vi "Calc Safe Reports.vi"(8 "tolerate 1 bad level?":bool, 9 "lower limit":i32, 10 "upper limit":i32, 11 "Reports":cluster{i32[]}[](array[cluster])) -> (3 "safe reports":u32)   [LabVIEW 2020, in "AoC 2024.lvlib"]
uses:
  AoC 2024.lvlib
panel:
  out "Analysed Reports":cluster{i32[], i32[], bool, "Digit":i32}[](array[cluster])
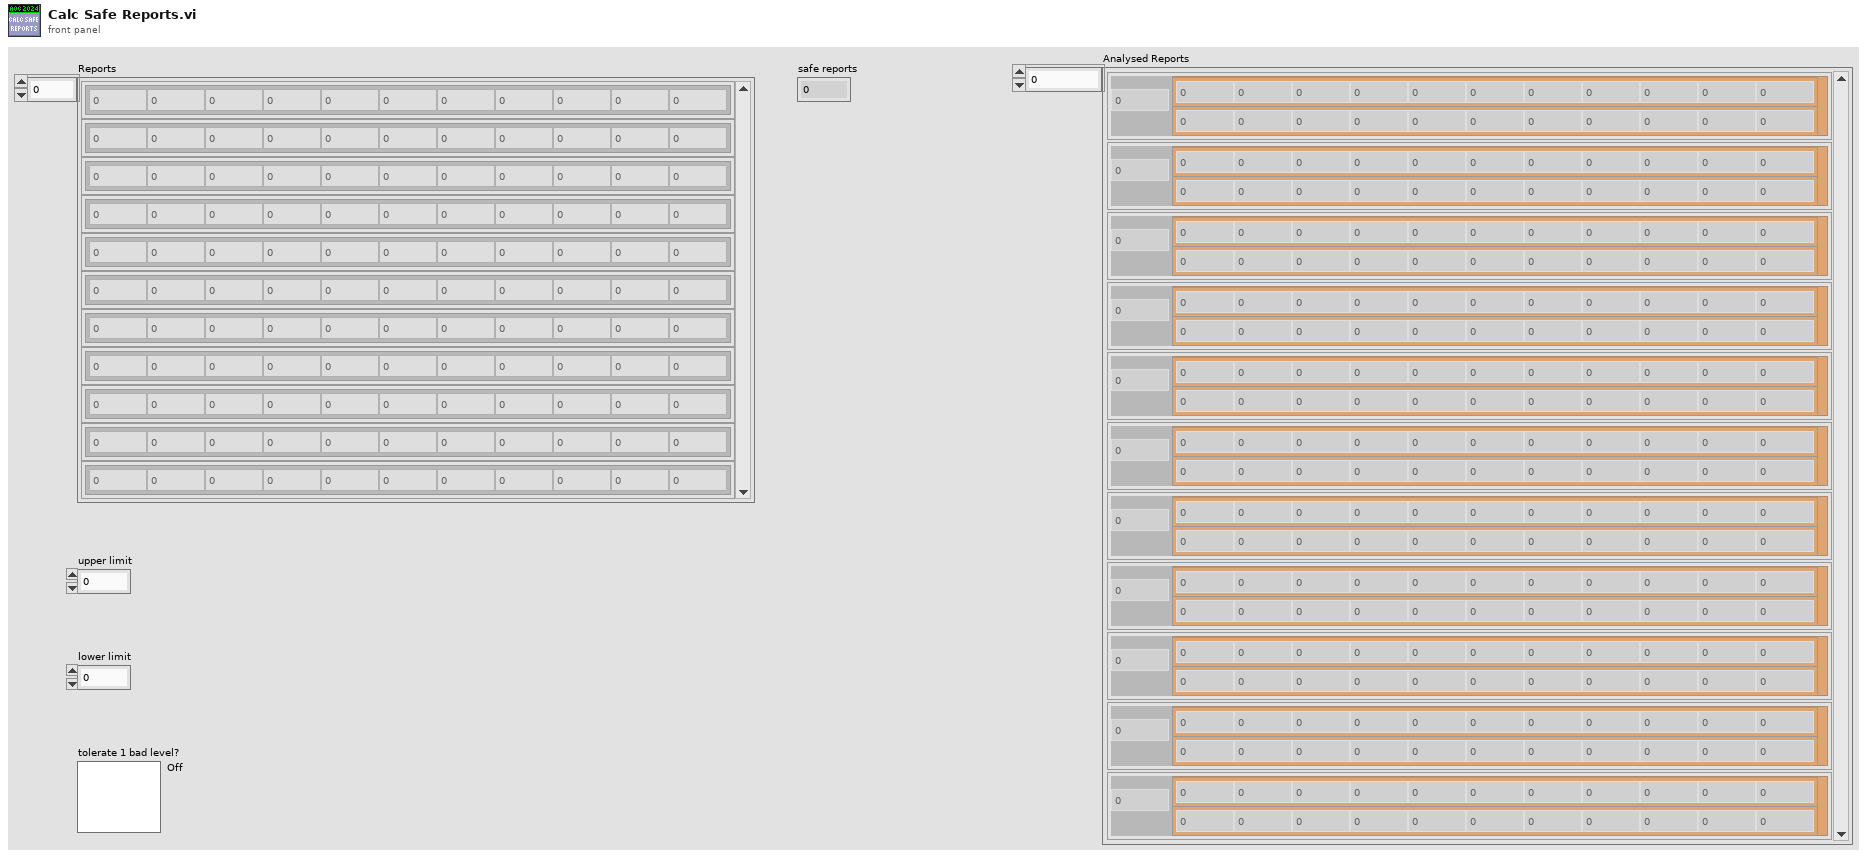
[diagram p1: front panel]
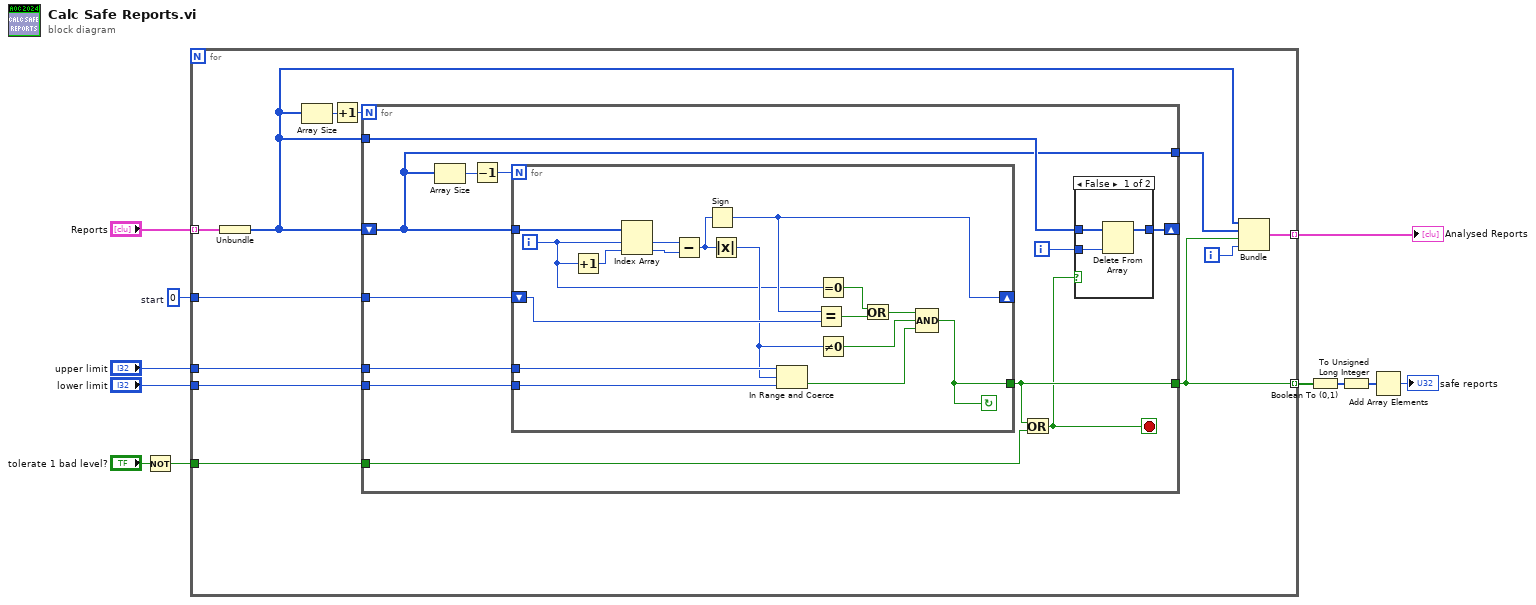
[diagram p0: block diagram]
diagram:
  w11 = 0  # start
  n1 = Not(x="tolerate 1 bad level?") -> (.not. x?=w5:bool)
  n2 = for {
    tunnel: "Reports" -> [w20] mode=indexing
    tunnel: "upper limit" -> [w23]
    tunnel: "lower limit" -> [w22]
    tunnel: w11 -> [w21]
    tunnel: w5 -> [w19]
    tunnel: [w16] -> w4 mode=indexing
    tunnel: [w18] -> w10 mode=indexing
    i -> [w17]
    n3 = Unbundle(w20) -> (w15:i32[])
    n4 = Array Size(array=w15) -> (size(s)=w14:i32)
    n5 = Increment(x=w14) -> (x+1=w13:i32)
    n6 = for {
      N: w13 -> [_]
      tunnel: w23 -> [w35]
      tunnel: w22 -> [w34]
      tunnel: w21 -> [w33]
      tunnel: [w30] -> w18
      shift-right: [w29] -> _
      shift-left: w15 -> [w24]
      tunnel: w19 -> [w27]
      tunnel: w15 -> [w25]
      tunnel: [w24] -> w12
      i -> [w28]
      stop <- w26 stop-if-true
      n7 = Array Size(array=w24) -> (size(s)=w32:i32)
      n8 = Decrement(x=w32) -> (x-1=w31:i32)
      n9 = for {
        N: w31 -> [_]
        tunnel: w24 -> [w56]
        tunnel: w35 -> [w53]
        tunnel: w34 -> [w52]
        tunnel: [w47] -> w30
        shift-right: [w50] -> _
        shift-left: w33 -> [w45]
        i -> [w43]
        stop <- w47 continue-if-true
        n10 = Increment(x=w43) -> (x+1=w41:i32)
        n11 = Index Array(array=w56, index #1=w43, index #2=w41) -> (element #1=w55:i32, element #2=w54:i32)
        n12 = Subtract(x=w55, y=w54) -> (x-y=w51:i32)
        n13 = Sign(1:w51) -> (0:w50:i32)
        n14 = Absolute Value(x=w51) -> (abs(x)=w44:i32)
        n15 = In Range and Coerce(upper limit=w53, x=w44, lower limit=w52) -> (In Range?=w48:bool)  [unwired: 1 out]
        n16 = Equal?(x=w50, y=w45) -> (x = y?=w49:bool)
        n17 = Equal To 0?(x=w43) -> (x = 0?=w40:bool)
        n18 = Not Equal To 0?(x=w44) -> (x != 0?=w42:bool)
        n19 = Or(x=w40, y=w49) -> (x .or. y?=w46:bool)
        n20 = Compound Arithmetic op=AND(w46, w42, w48) -> (w47:bool)
      }
      n21 = Or(x=w30, y=w27) -> (x .or. y?=w26:bool)
      n22 = case shown="False" w26 {
        tunnel: w25 -> [w38 w39]
        tunnel: [w37 w39] -> w29
        tunnel: w28 -> [w36 _]
        frame False {
          n23 = Delete From Array(array=w38, index=w36) -> (array with subset deleted=w37:i32[])  [unwired: 1 in, 1 out]
        }
        frame True {
        }
      }
    }
    n24 = Bundle(w15, w12, w18, w17) -> (w16:cluster{i32[], i32[], bool, i32})  [unwired: 1 in]
  }
  "Analysed Reports" <- w4
  n25 = Boolean To (0,1)(Boolean=w10) -> (0, 1=w3:i16[])
  n26 = To Unsigned Long Integer(number=w3) -> (unsigned 32bit integer=w1:u32[])
  n27 = Add Array Elements(numeric array=w1) -> (sum=→"safe reports":u32)
